vi "Cheesy Color Scoring.vi"(5 "ROI Out":T2[](array[typedef]) {"Contours"."Type" items=["No Selection", "Point", "Line", "Rectangle", "Oval", "Polygon", "Freehand Region", "Annulus", "Unused2", "Unused3", "Broken Line", "Freehand Line", "Rotated Rectangle"]}, 6 "Threshold":sgl, 8 "error in (no error)":errorcluster, 9 "Source Image In":T1) -> (1 "ROI Different":bool[](array[boolean]), 2 "ROI Scores":sgl[](array[numeric]), 3 "Source Image Out":T1)   [LabVIEW 2015]
uses:
  <vilib>/vision/Image Controls.llb/IMAQ Image.ctl
  <vilib>/vision/NI_Vision_Development_Module.lvlib
panel:
  out "Val Chart":T3(graph)
  out "Sat Chart":T3(graph)
  out "Hue Chart":T3(graph)
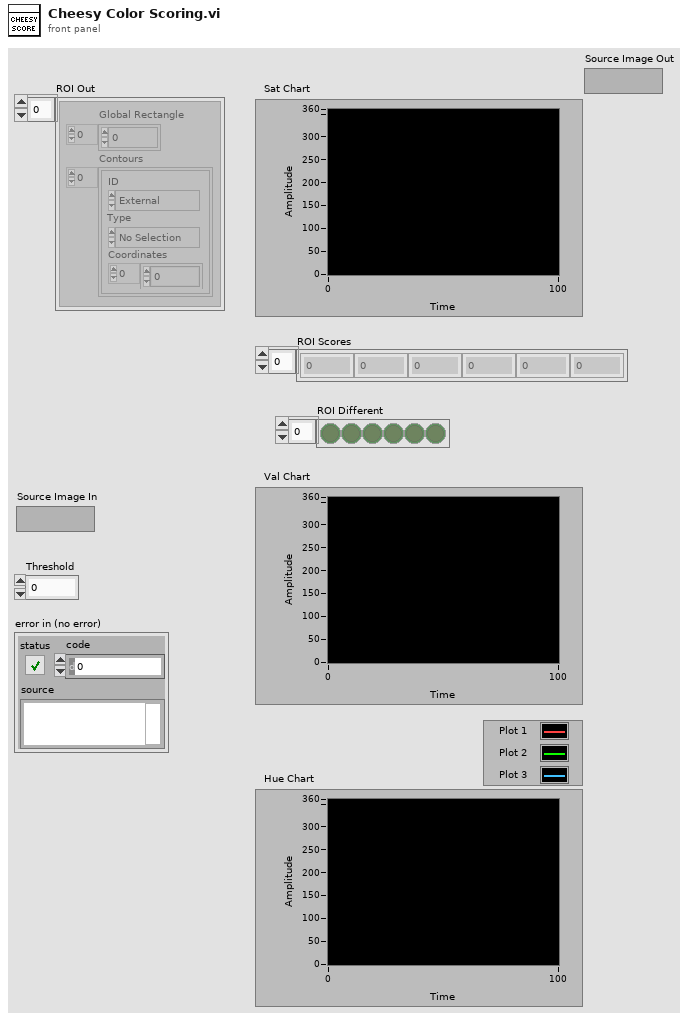
[diagram p1: front panel]
types:
  T1 = typedef "IMAQ Image.ctl" = refnum<image>
  T2 = typedef "ROI Descriptor" = cluster{"Global Rectangle":i32[], "Contours":cluster{"ID":enum32{"External", "Internal"}, "Type":u32, "Coordinates":i32[]}[]}
  T3 = cluster{"[0]":sgl, "[1]":sgl, "[2]":sgl, "[3]":sgl}
  T4 = typedef "Image Type" = u32
  T5 = cluster{"Min":sgl, "Max":sgl, "Mean":sgl, "Std Dev":sgl, "Count":i32}
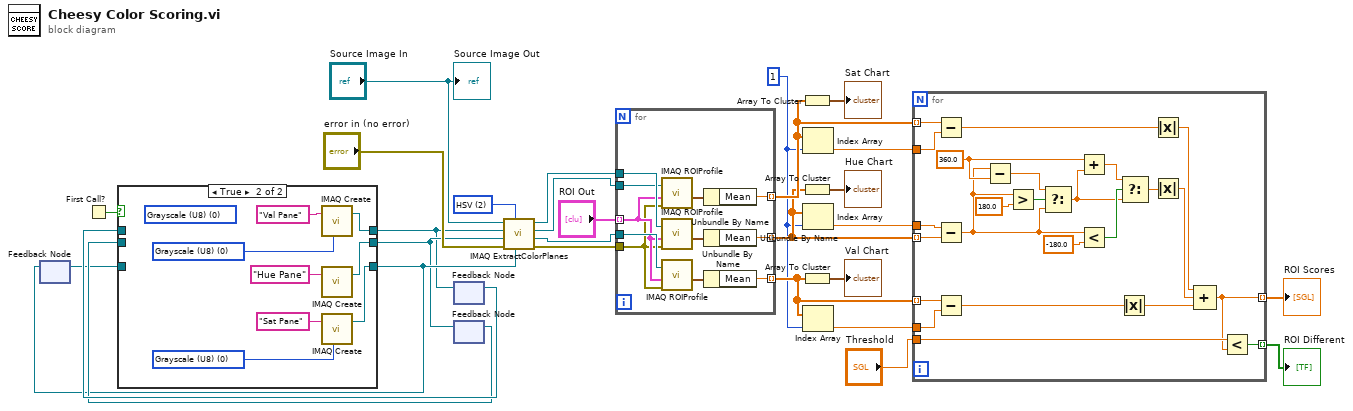
[diagram p0: block diagram]
diagram:
  w17 = 1 ("index")
  w11 = u16 2 items=["RGB", "HSL", "HSV", "HSI"] ("Color Mode")
  n1 = feedback #1() -> (w4:T1)  [unwired: 1 in]
  n2 = First Call?() -> (First Call?: T/F=w7:bool)
  n3 = feedback #2() -> (w6:T1)  [unwired: 1 in]
  n4 = feedback #3() -> (w5:T1)  [unwired: 1 in]
  n5 = case shown="True" w7 {
    tunnel: [w29 w37] -> w3
    tunnel: [w30 w35] -> w2
    tunnel: [w31 w32] -> w1
    tunnel: w6 -> [w31 _]
    tunnel: w5 -> [w30 _]
    tunnel: w4 -> [w29 _]
    frame False {
    }
    frame True {
      w33 = T4 0 items=["Grayscale (U8)", "Grayscale (I16)", "Grayscale (SGL)", "Complex (CSG)", "RGB (U32)", "HSL (U32)", "RGB (U64)", "Grayscale (U16)"] ("Image Type")
      (unwired) T4 0 items=["Grayscale (U8)", "Grayscale (I16)", "Grayscale (SGL)", "Complex (CSG)", "RGB (U32)", "HSL (U32)", "RGB (U64)", "Grayscale (U16)"] ("Image Type")
      w39 = T4 0 items=["Grayscale (U8)", "Grayscale (I16)", "Grayscale (SGL)", "Complex (CSG)", "RGB (U32)", "HSL (U32)", "RGB (U64)", "Grayscale (U16)"] ("Image Type")
      n6 = call "IMAQ Create"("Image Name"="Val Pane", "Image Type"=w33) -> ("New Image"=w32:T1)  [unwired: 2 in, 2 out]
      n7 = call "IMAQ Create"("Image Name"="Hue Pane") -> ("New Image"=w35:T1)  [unwired: 3 in, 2 out]
      n8 = call "IMAQ Create"("Image Name"="Sat Pane", "Image Type"=w39) -> ("New Image"=w37:T1)  [unwired: 2 in, 2 out]
    }
  }
  n9 = feedback-in #1(w3) -> ()
  n10 = feedback-in #2(w1) -> ()
  n11 = feedback-in #3(w2) -> ()
  n12 = call "IMAQ ExtractColorPlanes"("Blue or Luma or Val or Inten Plane"=w3, "Color Mode"=w11, "error in (no error)"="error in (no error)", "Green or Sat Plane"=w2, "Red or Hue Plane"=w1, "Image Src"="Source Image In") -> ("error out"=w13:errorcluster, "Blue or Luma or Val or Inten Plane out"=w16:T1, "Green or Sat Plane out"=w15:T1, "Red or Hue Plane out"=w12:T1)  [unwired: 2 in]
  n13 = for {
    tunnel: "ROI Out" -> [w45] mode=indexing
    tunnel: w13 -> [w44]
    tunnel: w12 -> [w50]
    tunnel: [w48] -> w18 mode=indexing
    tunnel: w15 -> [w47]
    tunnel: w16 -> [w46]
    tunnel: [w41] -> w26 mode=indexing
    tunnel: [w40] -> w27 mode=indexing
    n14 = call "IMAQ ROIProfile"("error in (no error)"=w44, "ROI Descriptor"=w45, "Image"=w47) -> ("ROI Pixel Statistics"=w43:T5)  [unwired: 1 in, 4 out]
    n15 = call "IMAQ ROIProfile"("error in (no error)"=w44, "ROI Descriptor"=w45, "Image"=w50) -> ("ROI Pixel Statistics"=w49:T5)  [unwired: 1 in, 4 out]
    n16 = call "IMAQ ROIProfile"("error in (no error)"=w44, "ROI Descriptor"=w45, "Image"=w46) -> ("ROI Pixel Statistics"=w42:T5)  [unwired: 1 in, 4 out]
    n17 = Unbundle By Name(w43) -> ("Mean"=w41:sgl)
    n18 = Unbundle By Name(w49) -> ("Mean"=w48:sgl)
    n19 = Unbundle By Name(w42) -> ("Mean"=w40:sgl)
  }
  n20 = Array To Cluster(array=w26) -> (cluster=→"Sat Chart":T3)
  n21 = Array To Cluster(array=w18) -> (cluster=→"Hue Chart":T3)
  n22 = Array To Cluster(array=w27) -> (cluster=→"Val Chart":T3)
  n23 = Index Array(array=w26, index=w17) -> (element=w20:sgl)
  n24 = Index Array(array=w18, index=w17) -> (element=w19:sgl)
  n25 = Index Array(array=w27, index=w17) -> (element=w21:sgl)
  n26 = for {
    tunnel: w18 -> [w66] mode=indexing
    tunnel: w19 -> [w74]
    tunnel: w26 -> [w63] mode=indexing
    tunnel: w20 -> [w64]
    tunnel: w27 -> [w62] mode=indexing
    tunnel: w21 -> [w61]
    tunnel: "Threshold" -> [w54]
    tunnel: [w53] -> w23 mode=indexing
    tunnel: [w52] -> w28 mode=indexing
    w65 = sgl 360.0 ("x")
    n27 = Subtract(x=w63, y=w64) -> (x-y=w60:sgl)
    n28 = Subtract(x=w74, y=w66) -> (x-y=w51:sgl)
    n29 = Subtract(x=w62, y=w61) -> (x-y=w59:sgl)
    n30 = Subtract(x=w51, y=w65) -> (x-y=w67:sgl)
    n31 = Greater?(x=w51, y=sgl 180.0) -> (0:w70:bool)
    n32 = Select(t=w67, s=w70, f=w51) -> (s? t:f=w68:sgl)
    n33 = Add(x=w65, y=w68) -> (x+y=w69:sgl)
    n34 = Less?(x=w51, y=sgl -180.0) -> (x < y?=w71:bool)
    n35 = Absolute Value(x=w59) -> (abs(x)=w55:sgl)
    n36 = Select(t=w69, s=w71, f=w68) -> (s? t:f=w58:sgl)
    n37 = Absolute Value(x=w60) -> (abs(x)=w57:sgl)
    n38 = Absolute Value(x=w58) -> (abs(x)=w56:sgl)
    n39 = Compound Arithmetic op=ADD(w57, w56, w55) -> (w52:sgl)
    n40 = Less?(x=w54, y=w52) -> (x < y?=w53:bool)
  }
  "ROI Scores" <- w28
  "ROI Different" <- w23
  "Source Image Out" <- "Source Image In"
